vi "MeasureFilterIntensities.vi"(11 "Ctl Refnum":refnum<vi>) -> ()   [LabVIEW 2011]
uses:
  <vilib>/Utility/file.llb/Write To Spreadsheet File (DBL).vi
panel:
  in  "Current Angle (degrees)":dbl
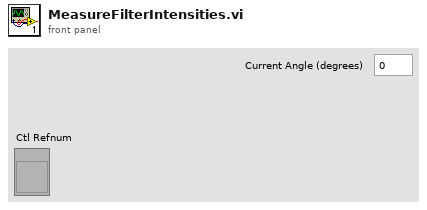
[diagram p1: front panel]
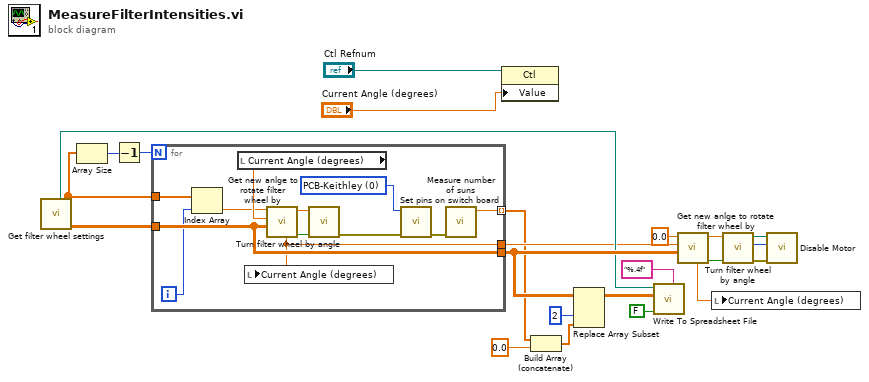
[diagram p0: block diagram]
diagram:
  n1 = call "Get filter wheel settings.vi"() -> ("All filter wheel settings"=w15:dbl[][], "Filter wheel numbers"=w8:dbl[], "Filter wheel settings file path"=w16:path)  [unwired: 7 in, 2 out]
  n2 = Array Size(array=w8) -> (size(s)=w10:i32)
  n3 = Decrement(x=w10) -> (x-1=w9:i32)
  n4 = for {
    N: w9 -> [_]
    tunnel: w15 -> [w32]
    tunnel: [w33] -> w5 mode=indexing
    tunnel: [w32] -> w22
    tunnel: [w27] -> w11
    tunnel: w8 -> [w24]
    i -> [w25]
    w28 = u16 0 items=["PCB-Keithley", "PCB-EQE", "Manual-Keithley", "Manual-EQE"] ("Experiment type")
    n5 = Index Array(array=w24, index=w25) -> (element=w26:dbl)
    n6 = local read "Current Angle (degrees)"() -> (w31:dbl)
    n7 = call "Get new anlge to rotate filter wheel by.vi"("Filter Wheel Positions"=w32, "Current anlge (degrees)"=w31, "Filter no."=w26) -> ("Clockwise?"=w34:bool, "Rotate by angle (degrees)"=w35:dbl, "New current anlge (degrees)"=w27:dbl)  [unwired: 6 in]
    n8 = local write "Current Angle (degrees)"(w27) -> ()
    n9 = call "Turn filter wheel by angle.vi"("Clockwise?"=w34, "Angle (degrees)"=w35) -> ("error out"=w30:errorcluster)  [unwired: 7 in, 2 out]
    n10 = call "Set pins on switch board.vi"("Error In"=w30, "Experiment type"=w28) -> ("error out"=w29:errorcluster)  [unwired: 9 in]
    n11 = call "Measure number of suns.vi"("error in (no error)"=w29) -> ("Number of suns"=w33:dbl)  [unwired: 9 in, 1 out]
  }
  n12 = property class="Ctl"(reference="Ctl Refnum", "Value"="Current Angle (degrees)") -> ()  [unwired: 1 in, 2 out]
  n13 = Build Array (concatenate)(w5, 0.0 ("Filter no.")) -> (w6:dbl[])
  n14 = Replace Array Subset(array=w22, new element=w6, index (col)=2 ("disabled index (col)")) -> (w23:dbl[][])  [unwired: 1 in]
  n15 = call-poly <vilib>:"Write To Spreadsheet File.vi"("format (%.3f)"="%.4f", "append to file? (new file:F)"=FALSE, "2D data"=w23, "file path (dialog if empty)"=w16) -> ()  [unwired: 4 in, 1 out]
  n16 = call "Get new anlge to rotate filter wheel by.vi"("Filter Wheel Positions"=w22, "Current anlge (degrees)"=w11, "Filter no."=0.0) -> ("Clockwise?"=w20:bool, "Rotate by angle (degrees)"=w21:dbl, "New current anlge (degrees)"=w14:dbl)  [unwired: 6 in]
  n17 = local write "Current Angle (degrees)"(w14) -> ()
  n18 = call "Turn filter wheel by angle.vi"("Clockwise?"=w20, "Angle (degrees)"=w21) -> ("error out"=w12:errorcluster, "Enable Channel out"=w18:u8, "Serial Port out"=w19:refnum<visa-resource-name>)  [unwired: 7 in]
  n19 = call "Disable Motor.vi"("Error In"=w12, "Enable Channel"=w18, "Serial Port"=w19) -> ()  [unwired: 8 in, 1 out]
